vi "ExtendedRegisterReadLong.vi"(6 "Compare Bits In":T1[](array[typedef]) {"Expected Value(s)" format="%.0x"}, 7 "Extended Read/Write Long":T2 {"Data" format="%.0x"; "Register" format="%.0x"; "Slave Address" max=15 format="%.0x"}, 8 "error in (no error)":errorcluster, 9 "Number of Samples In":i32, 10 "Data Array":u8[][](array[numeric]), 11 "RFFE_Data In":T3 {"Toggle (high to low)" items=["0", "1", "Z", "L", "H", "X", "T", "V"]; "X Array" items=["0", "1", "Z", "L", "H", "X", "T", "V"]; "Z Array" items=["0", "1", "Z", "L", "H", "X", "T", "V"]; "L Array" items=["0", "1", "Z", "L", "H", "X", "T", "V"]; "H Array" items=["0", "1", "Z", "L", "H", "X", "T", "V"]; "One Array" items=["0", "1", "Z", "L", "H", "X", "T", "V"]; "Zero Array" items=["0", "1", "Z", "L", "H", "X", "T", "V"]}) -> (0 "error out":errorcluster, 1 "Number of Samples Out out":i32, 2 "Data Array Out":u8[][](array[numeric]), 3 "RFFE_Data Out":T3 {"Toggle (high to low)" items=["0", "1", "Z", "L", "H", "X", "T", "V"]; "X Array" items=["0", "1", "Z", "L", "H", "X", "T", "V"]; "Z Array" items=["0", "1", "Z", "L", "H", "X", "T", "V"]; "L Array" items=["0", "1", "Z", "L", "H", "X", "T", "V"]; "H Array" items=["0", "1", "Z", "L", "H", "X", "T", "V"]; "One Array" items=["0", "1", "Z", "L", "H", "X", "T", "V"]; "Zero Array" items=["0", "1", "Z", "L", "H", "X", "T", "V"]}, 4 "Compare Bits Out":T1[](array[typedef]) {"Expected Value(s)" format="%.0x"})   [LabVIEW 2011]
doc: "Builds MIPI RFFE Extended Register Read Long with the specified data."
uses:
  Ctrls/RFFE_Data.ctl
  Ctrls/ClockDataChannels.ctl
  Ctrls/ExtendedRegReadWriteLong.ctl
  Ctrls/ReadInfo.ctl
  Ctrls/Commands.ctl
  Ctrls/Read_Write_Data.ctl
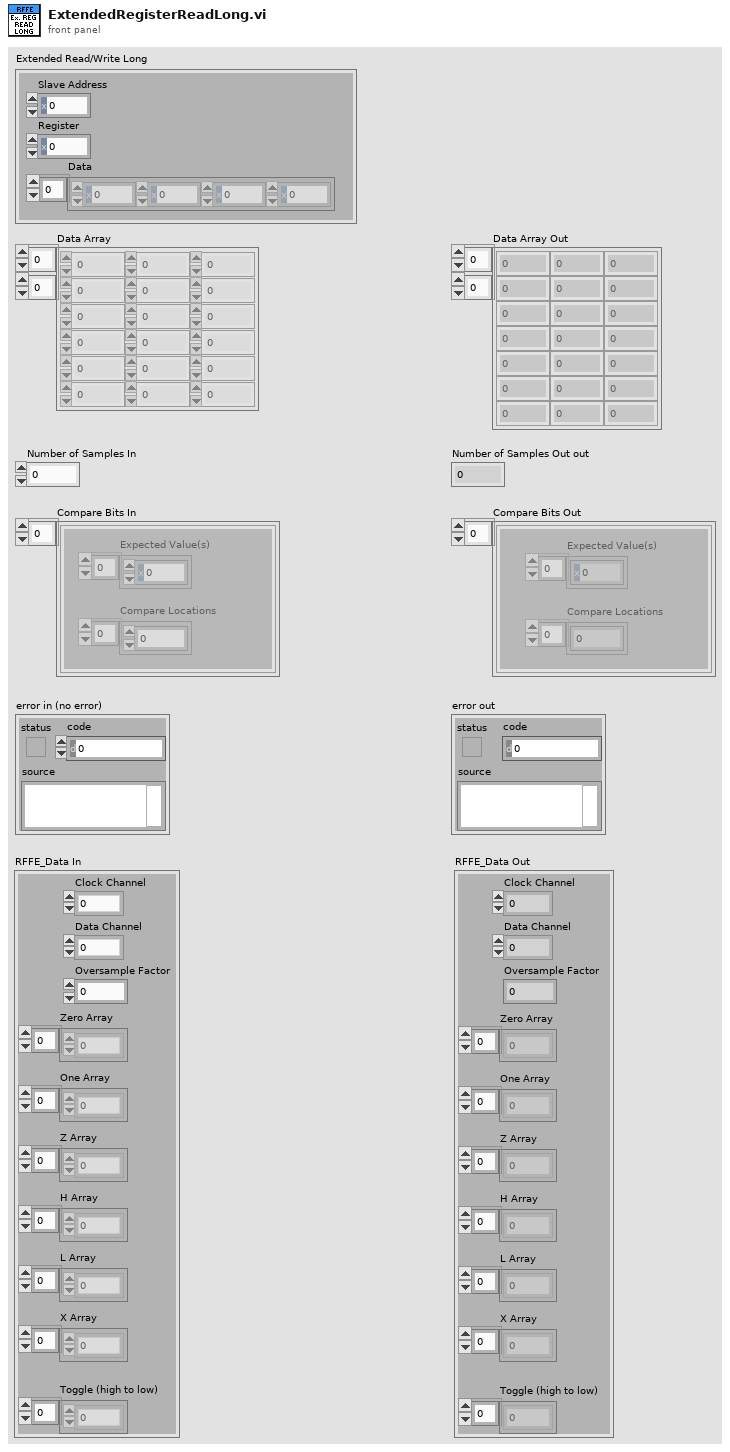
[diagram p1: front panel]
types:
  T1 = typedef "ReadInfo.ctl" = cluster{"Expected Value(s)":u8[], "Compare Locations":u32[]}
  T2 = typedef "ExtendedRegReadWriteLong.ctl" = cluster{"Slave Address":u8, "Register":u16, "Data":u8[]}
  T3 = typedef "RFFE_Data.ctl" = cluster{"Clock Channel":T4, "Data Channel":T4, "Oversample Factor":u8, "Zero Array":u8[], "One Array":u8[], "Z Array ":u8[], "H Array":u8[], "L Array":u8[], "X Array":u8[], "Toggle (high to low)":u8[]}
  T4 = typedef "ClockDataChannels.ctl" = enum16{"0", "1"}
  T5 = typedef "Read_Write_Data.ctl" = cluster{"Data":u8, "Read/Write":enum16{"Read", "Write"}}
  T6 = typedef "Commands.ctl" = cluster{"Command":enum16{"Extended Register Write", "Extended Register Read", "Extended Register Write Long", "Extended Register Read Long", "Register Write", "Register Read", "Register 0 Write"}, "Data/Address/ByteCount":u8}
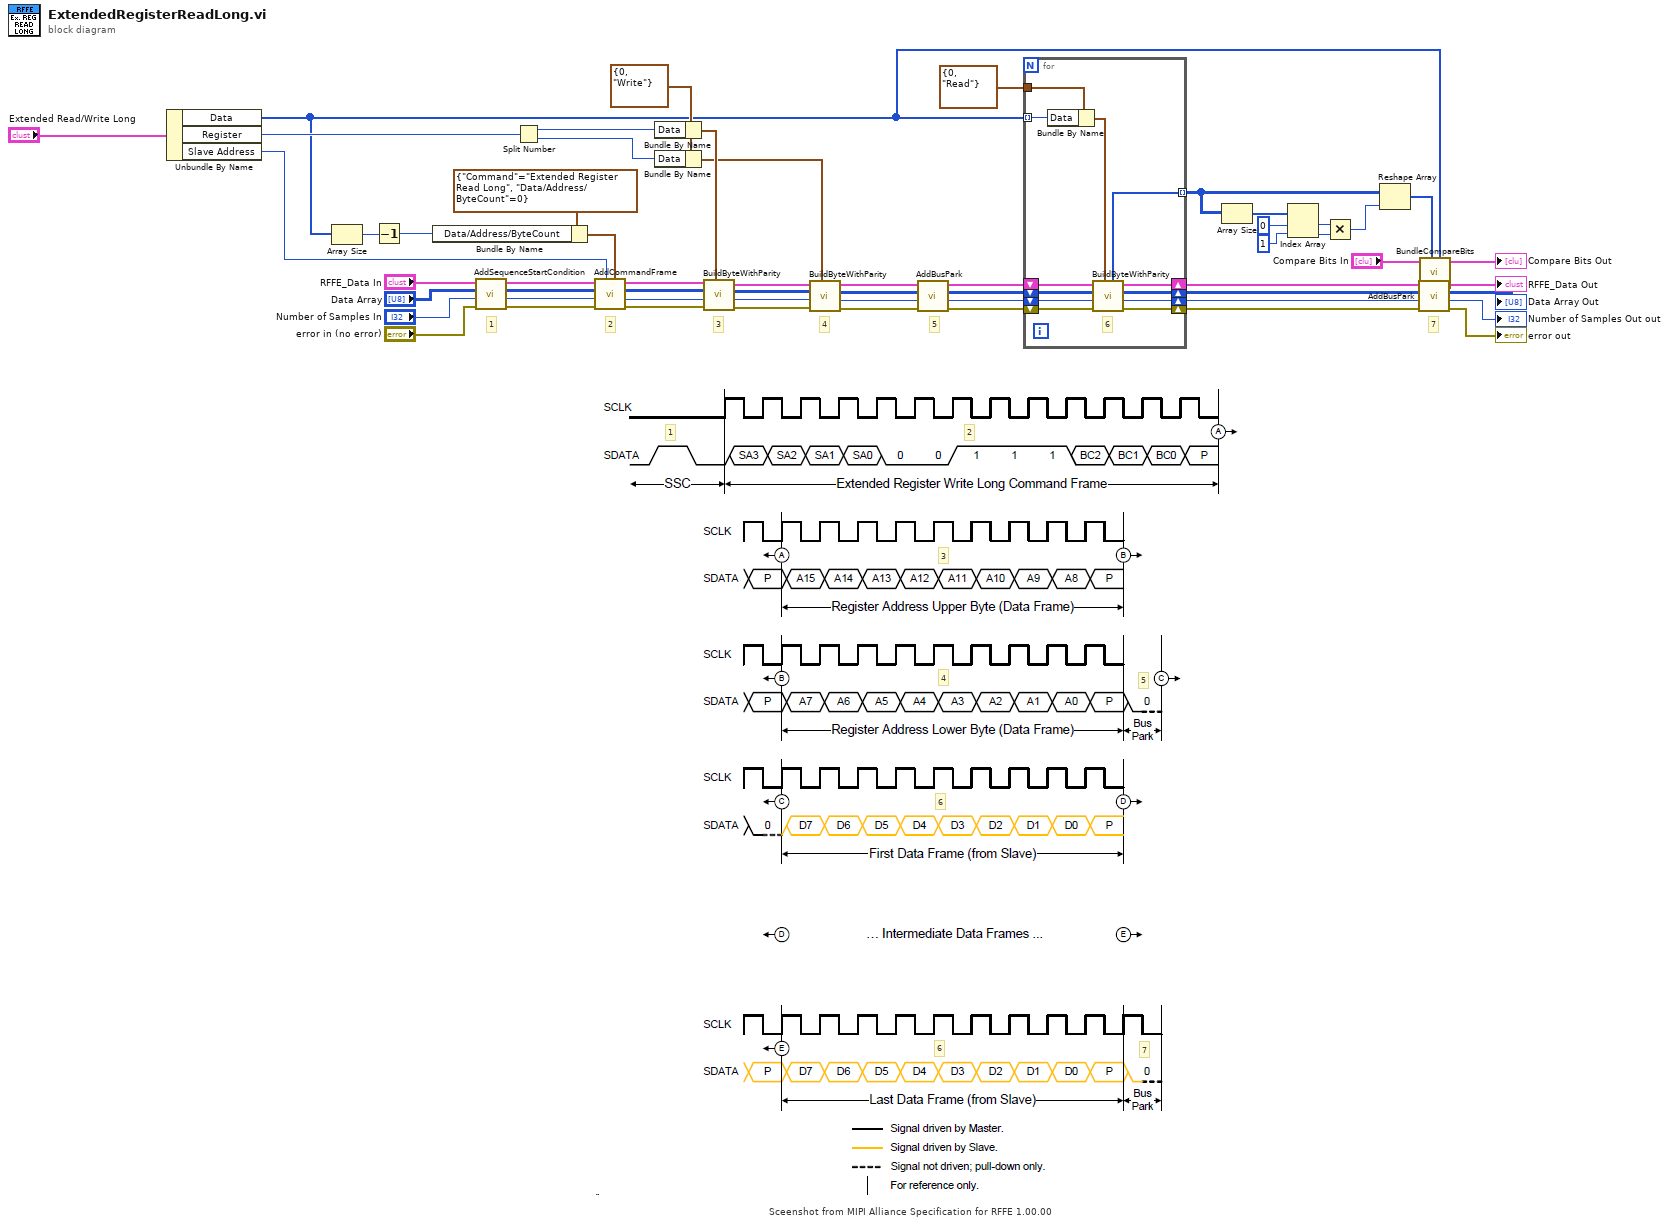
[diagram p0: block diagram]
diagram:
  w32 = T5 {"Data"=0, "Read/Write"=enum."Write"} ("Read/Write Data")
  # "Sceenshot from MIPI Alliance Specification for RFFE 1.00.00"
  # "6"
  # "7"
  # "6"
  # "5"
  # "4"
  # "3"
  # "2"
  # "1"
  # "7"
  # "5"
  # "4"
  # "3"
  # "2"
  # "1"
  n1 = Unbundle By Name("Extended Read/Write Long") -> ("Data"=w4:u8[], "Register"=w34:u16, "Slave Address"=w13:u8)
  n2 = Array Size(array=w4) -> (size(s)=w35:i32)
  n3 = Decrement(x=w35) -> (x-1=w24:i32)
  n4 = Bundle By Name(cluster=T6 {"Command"=enum."Extended Register Read Long", "Data/Address/ByteCount"=0} ("Command"), "Data/Address/ByteCount"=w24) -> (w14:T6)
  n5 = call "AddSequenceStartCondition.vi"("error in (no error)"="error in (no error)", "Number of Samples In"="Number of Samples In", "Data Array In"="Data Array", "RFFE_Data In"="RFFE_Data In") -> ("error out"=w46:errorcluster, "Number of Samples Out"=w54:i32, "Data Array Out"=w47:u8[][], "RFFE_Data Out"=w48:T3)  [unwired: 4 in]
  n6 = Split Number(x=w34) -> (hi(x)=w33:u8, lo(x)=w31:u8)
  n7 = call "AddCommandFrame.vi"("Command"=w14, "Slave Address"=w13, "error in (no error)"=w46, "Number of Samples In"=w54, "Data Array In"=w47, "RFFE_Data"=w48) -> ("error out"=w49:errorcluster, "Number of Samples Out"=w51:i32, "Data Array Out"=w52:u8[][], "Configuratation Out"=w50:T3)  [unwired: 2 in]
  n8 = Bundle By Name(cluster=w32, "Data"=w33) -> (w26:T5)
  n9 = Bundle By Name(cluster=w32, "Data"=w31) -> (w25:T5)
  n10 = call "BuildByteWithParity.vi"("Read/Write Data"=w26, "error in"=w49, "Number of Samples In"=w51, "Data Array In"=w52, "RFFE_Data In"=w50) -> ("error out"=w30:errorcluster, "Number of Samples Out"=w29:i32, "Data Array Out"=w28:u8[][], "RFFE_Data Out"=w27:T3)  [unwired: 2 in, 1 out]
  n11 = call "BuildByteWithParity.vi"("Read/Write Data"=w25, "error in"=w30, "Number of Samples In"=w29, "Data Array In"=w28, "RFFE_Data In"=w27) -> ("error out"=w22:errorcluster, "Number of Samples Out"=w17:i32, "Data Array Out"=w20:u8[][], "RFFE_Data Out"=w16:T3)  [unwired: 2 in, 1 out]
  n12 = call "AddBusPark.vi"("error in (no error)"=w22, "Number of Samples In"=w17, "Data Array In"=w20, "RFFE_Data In"=w16) -> ("error out"=w21:errorcluster, "Number of Samples Out"=w18:i32, "Data Array Out"=w19:u8[][], "RFFE_Data Out"=w15:T3)  [unwired: 4 in]
  n13 = for {
    shift-right: [w67] -> w38
    shift-left: w21 -> [w68]
    shift-right: [w64] -> w36
    shift-left: w18 -> [w66]
    shift-right: [w63] -> w37
    shift-left: w19 -> [w65]
    shift-right: [w62] -> w3
    shift-left: w15 -> [w61]
    tunnel: w4 -> [w60] mode=indexing
    tunnel: T5 {"Data"=0, "Read/Write"=enum."Read"} ("Read/Write Data") -> [w58]
    tunnel: [w57] -> w6 mode=indexing
    # "6"
    n14 = Bundle By Name(cluster=w58, "Data"=w60) -> (w59:T5)
    n15 = call "BuildByteWithParity.vi"("Read/Write Data"=w59, "error in"=w68, "Number of Samples In"=w66, "Data Array In"=w65, "RFFE_Data In"=w61) -> ("error out"=w67:errorcluster, "Number of Samples Out"=w64:i32, "Data Array Out"=w63:u8[][], "RFFE_Data Out"=w62:T3, "Compare Locations"=w57:u32[])  [unwired: 2 in]
  }
  n16 = Array Size(array=w6) -> (size(s)=w8:i32[])
  n17 = Index Array(array=w8, index #1=0 ("index"), index #2=1 ("index")) -> (element #1=w9:i32, element #2=w7:i32)
  n18 = Multiply(x=w9, y=w7) -> (x*y=w10:i32)
  n19 = Reshape Array(w6, w10) -> (w5:u32[])
  n20 = call "AddBusPark.vi"("error in (no error)"=w38, "Number of Samples In"=w36, "Data Array In"=w37, "RFFE_Data In"=w3) -> ("error out"=→"error out":errorcluster, "Number of Samples Out"=→"Number of Samples Out out":i32, "Data Array Out"=→"Data Array Out":u8[][], "RFFE_Data Out"=→"RFFE_Data Out":T3)  [unwired: 4 in]
  n21 = call "BundleCompareBits.vi"("Expected Value(s)"=w4, "Compare Locations"=w5, "Compare Bits In"="Compare Bits In") -> ("Compare Bits Out"=→"Compare Bits Out":T1[])  [unwired: 8 in]
